vi "Get_Position_Info.vi"(2 "Analysis Info cluster":T1[](array[typedef]) {"Sd Error in Variance" format="%.2f"; "Skew_u" format="%.2f"; "% u'/U" format="%.2f"; "Sd Error in Mean" format="%.2f"; "Kurt_u" format="%.2f"; "u^4" format="%.2f"; "u^3" format="%.2f"; "U" format="%.2f"; "u^2" format="%.2f"}, 3 "Setup file string":string) -> (0 "Analysis Info cluster 2":T1[](array[typedef]) {"Sd Error in Variance" format="%.2f"; "Skew_u" format="%.2f"; "% u'/U" format="%.2f"; "Sd Error in Mean" format="%.2f"; "Kurt_u" format="%.2f"; "u^4" format="%.2f"; "u^3" format="%.2f"; "U" format="%.2f"; "u^2" format="%.2f"})   [LabVIEW 2014]
uses:
  Controls/Analysis_info_cluster.ctl
  Controls/Inst_type.ctl
  Controls/Instrument_Array.ctl
  Controls/Post_Process.ctl
  Controls/User_Specific_mode.ctl
  Globals/Meas_global.vi
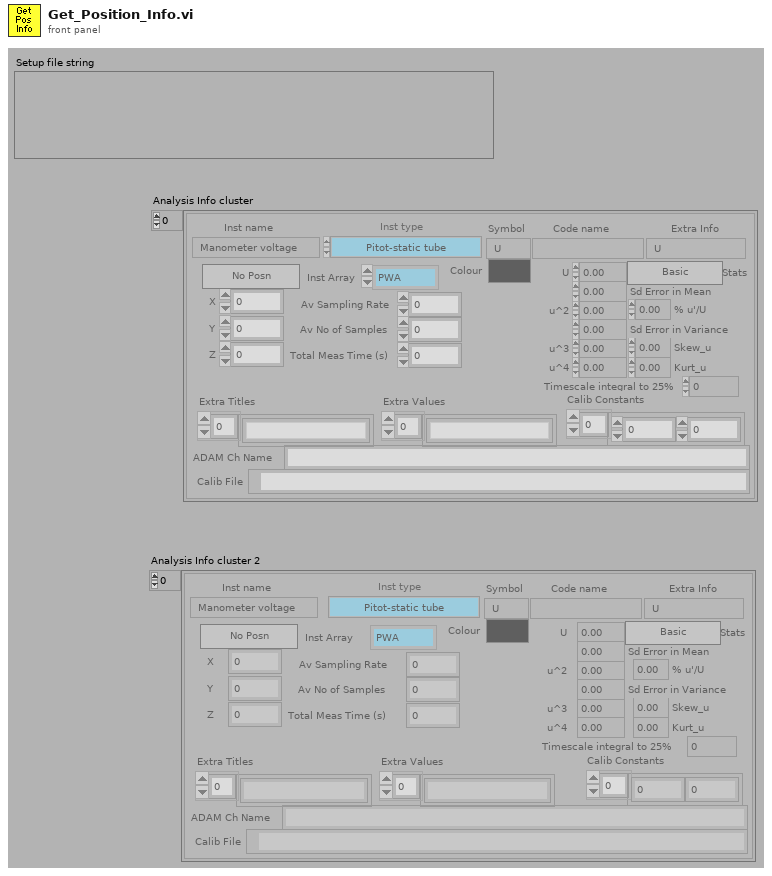
[diagram p1: front panel]
types:
  T1 = typedef "Analysis_info_cluster.ctl" = cluster{"Colour":u32, "Inst type":T2, "Inst name":string, "Symbol":string, "Code name":string, "Extra Info":string, "Inst Array":T3, "Extra Titles":string[], "Extra Values":string[], "U":dbl, "u^2":dbl, "u^3":dbl, "u^4":dbl, "Skew_u":dbl, "Kurt_u":dbl, "Sd Error in Mean":dbl, "% u'/U":dbl, "X":dbl, "Y":dbl, "Z":dbl, "Timescale integral to 25%":dbl, "Sd Error in Variance":dbl, "Calib File":path, "Calib Constants":dbl[], "Output Position":bool, "Full Stats":bool, "Av Sampling Rate":dbl, "Av No of Samples":dbl, "Total Meas Time (s)":dbl, "ADAM Ch Name":string}
  T2 = typedef "Inst_type.ctl" = enum16{"Propeller anemometer", "Raw voltage", "Pressure Transducer", "Pitot-static tube", "Preston tube", "Hot wire", "Cross wire 1", "Cross wire 2", "Generic Linear", "Generic Polynomial", "Generic BackPoly", "Fast FID", "Thermocouple", "Cold wire", "Pulsed Wire", "LDA Vel", "LDA Tran time", "LDA Arr time", "Microphone"}
  T3 = typedef "Instrument_Array.ctl" = enum16{"PWA", "LDA", "Analogue"}
  T4 = typedef "Post_Process.ctl" = enum16{"Take New Data", "Post Process Raw Data File"}
  T5 = typedef "User_Specific_mode.ctl" = enum16{"Check VI only", "Run VI"}
  T6 = cluster{"Values[0]":dbl, "Values[1]":dbl, "Values[2]":dbl}
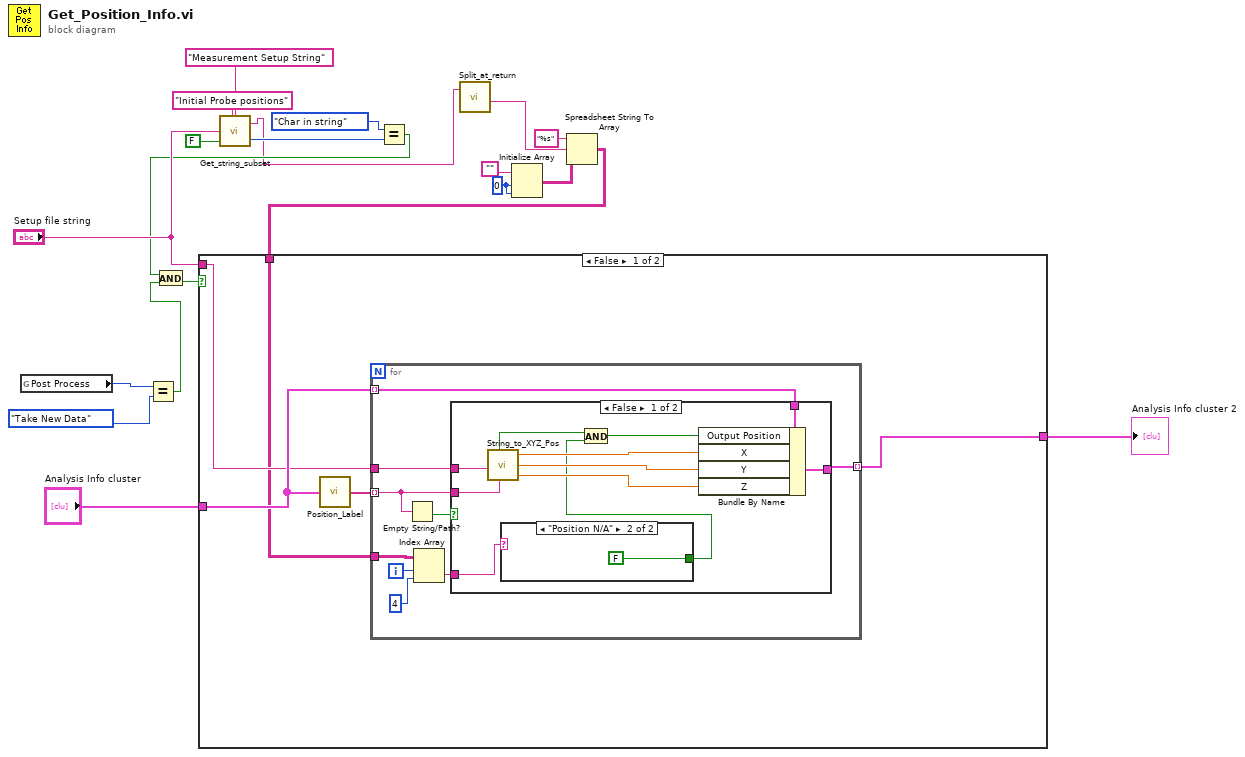
[diagram p0: block diagram]
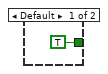
[diagram p2: hidden frame]
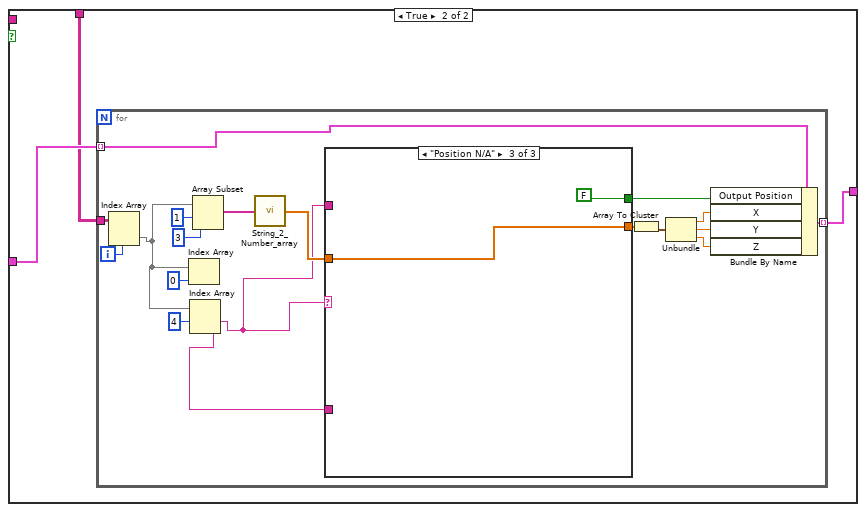
[diagram p4: hidden frame]
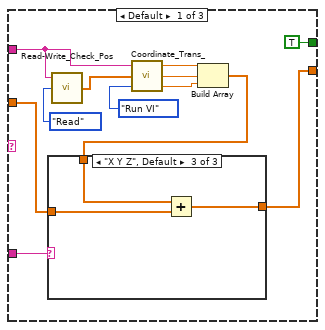
[diagram p5: hidden frame]
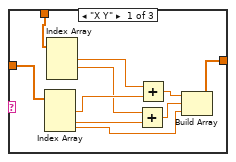
[diagram p6: hidden frame]
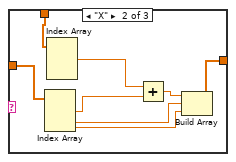
[diagram p7: hidden frame]
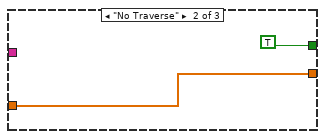
[diagram p8: hidden frame]
diagram:
  w4 = 0 ("Dimension Size")
  n1 = global read "Meas_global.vi" "Post Process"() -> (w20:T4)
  n2 = Equal?(x=w20, y=Post_Process."Take New Data" ("Post Process")) -> (x = y?=w10:bool)
  n3 = call "Get_string_subset.vi"("String Name"="Measurement Setup String", "Show Dialog?"=FALSE, "String to split"="Setup file string", "File Label"="Initial Probe positions") -> ("Status"=w14:enum16{"Char in string", "Char not in string"}, "Output string"=w2:string)
  n4 = Equal?(x=enum16{"Char in string", "Char not in string"}."Char in string" ("Status"), y=w14) -> (x = y?=w13:bool)
  n5 = And(x=w13, y=w10) -> (x .and. y?=w12:bool)
  n6 = call "Split_at_return.vi"("String"=w2) -> ("after substring"=w7:string)  [unwired: 1 in, 3 out]
  n7 = Initialize Array("", w4, w4) -> (w3:string[][])
  n8 = Spreadsheet String To Array(format string="%s", spreadsheet string=w7, array type (2D Dbl)=w3) -> (array=w1:string[][])  [unwired: 1 out]
  n9 = case shown="False" w12 {
    tunnel: "Setup file string" -> [w23 _]
    tunnel: "Analysis Info cluster" -> [w25 w51]
    tunnel: [w22 w50] -> w8
    tunnel: w1 -> [w21 w49]
    frame False {
      n10 = call "Position_Label.vi"("Analysis Info cluster"=w25) -> ("Position Label"=w24:string[])
      n11 = for {
        tunnel: w25 -> [w33] mode=indexing
        tunnel: [w34] -> w22 mode=indexing
        tunnel: w24 -> [w31] mode=indexing
        tunnel: w23 -> [w32]
        tunnel: w21 -> [w29]
        i -> [w28]
        n12 = Empty String/Path?(string/path=w31) -> (empty?=w30:bool)
        n13 = Index Array(array=w29, index (row)=w28, index (col)=4 ("index")) -> (element=w26:string)
        n14 = case shown="False" w30 {
          tunnel: [w45 w48] -> w34
          tunnel: w33 -> [w44 w48]
          tunnel: w31 -> [w43 _]
          tunnel: w32 -> [w42 _]
          tunnel: w26 -> [w37 _]
          frame False {
            n15 = call "String_to_XYZ_Pos.vi"("Input string"=w42, "Position label"=w43) -> ("Some labels found"=w36:bool, "X"=w41:dbl, "Y"=w40:dbl, "Z"=w39:dbl)  [unwired: 2 in]
            n16 = case shown="\"Position N/A\"" w37 {
              tunnel: [TRUE FALSE] -> w35
              frame Default {
              }
              frame "Position N/A" {
              }
            }
            n17 = And(x=w36, y=w35) -> (x .and. y?=w38:bool)
            n18 = Bundle By Name(cluster=w44, "Output Position"=w38, "X"=w41, "Y"=w40, "Z"=w39) -> (w45:T1)
          }
          frame True {
          }
        }
      }
    }
    frame True {
      n19 = for {
        tunnel: [w60] -> w50 mode=indexing
        tunnel: w51 -> [w58] mode=indexing
        tunnel: w49 -> [w56]
        i -> [w57]
        n20 = Index Array(array=w56, index (row)=w57) -> (element=w55:string[])  [unwired: 1 in]
        n21 = Index Array(array=w55, index=0) -> ()  [unwired: 1 out]
        n22 = Index Array(array=w55, index #1=4 ("index")) -> (element #1=w53:string, element #2=w54:string)  [unwired: 1 in]
        n23 = Array Subset(array=w55, index=1, length=3) -> (w59:string[])
        n24 = call "String_2_Number_array.vi"("Input String"=w59) -> ("Values"=w67:dbl[])
        n25 = case shown="\"Position N/A\"" w53 {
          tunnel: [w81 w105 w107] -> w68
          tunnel: w67 -> [w82 w105 w107]
          tunnel: w53 -> [w75 _ _]
          tunnel: w54 -> [w72 _ _]
          tunnel: [TRUE TRUE FALSE] -> w52
          frame Default {
            n26 = call "Read-Write_Check_Pos.vi"("Mode"=enum16{"Read", "Write"}."Read", "Traverse Name"=w75) -> ("Position Output"=w74:sgl[])  [unwired: 1 in]
            n27 = call "Coordinate_Trans_.vi"("Simulate/Run"=User_Specific_mode."Run VI", "Input Position"=w74, "Traverse Name"=w75) -> ("Z"=w78:dbl, "Y"=w79:dbl, "X"=w80:dbl)
            n28 = Build Array(w80, w79, w78) -> (w77:dbl[])
            n29 = case shown="\"X Y Z\", Default" w72 {
              tunnel: w82 -> [w92 w100 w103]
              tunnel: [w88 w96 w102] -> w81
              tunnel: w77 -> [w91 w99 w101]
              frame "X Y" {
                n30 = Index Array(array=w92) -> (element #1=w89:dbl, element #2=w85:dbl, element #3=w83:dbl)  [unwired: 3 in]
                n31 = Index Array(array=w91) -> (element #1=w90:dbl, element #2=w86:dbl)  [unwired: 3 in, 1 out]
                n32 = Add(x=w86, y=w85) -> (x+y=w84:dbl)
                n33 = Add(x=w90, y=w89) -> (x+y=w87:dbl)
                n34 = Build Array(w87, w84, w83) -> (w88:dbl[])
              }
              frame "X" {
                n35 = Index Array(array=w100) -> (element #1=w97:dbl, element #2=w93:dbl, element #3=w94:dbl)  [unwired: 3 in]
                n36 = Index Array(array=w99) -> (element #1=w98:dbl)  [unwired: 3 in, 2 out]
                n37 = Add(x=w98, y=w97) -> (x+y=w95:dbl)
                n38 = Build Array(w95, w93, w94) -> (w96:dbl[])
              }
              frame "X Y Z", Default {
                n39 = Add(x=w101, y=w103) -> (x+y=w102:dbl[])
              }
            }
          }
          frame "No Traverse" {
          }
          frame "Position N/A" {
          }
        }
        n40 = Array To Cluster(array=w68) -> (cluster=w66:T6)
        n41 = Unbundle(w66) -> ("Values[0]"=w65:dbl, "Values[1]"=w64:dbl, "Values[2]"=w63:dbl)
        n42 = Bundle By Name(cluster=w58, "Output Position"=w52, "X"=w65, "Y"=w64, "Z"=w63) -> (w60:T1)
      }
    }
  }
  "Analysis Info cluster 2" <- w8
